vi "DynamicDispatchJsonConstants.vi"() -> ()   [LabVIEW 2017, in "SubVIConverter.lvclass"]
uses:
  SubVIConverter.lvclass
panel:
  in  "HierarchyKey":string="Hierarchy"
  in  "NearestImplementationKey":string="Nearest"
  in  "ImplementationsKey":string="Implementations"
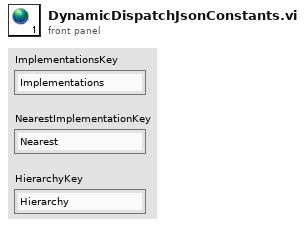
[diagram p1: front panel]
diagram:
